vi "VDD over Temp.vi"() -> ()   [LabVIEW 2020]
panel:
  out "Histeresis":dbl[](array[numeric])
  out "VDD down":dbl[](array[numeric])
  out "VDD up":dbl[](array[numeric])
  in  "Thermostream":refnum<visa-resource-name>="GPIB0::11::INSTR"
  out "error out":errorcluster
  in  "Multimetru":refnum<visa-resource-name>="GPIB0::24::INSTR"
  in  "SMU":refnum<visa-resource-name>="GPIB0::1::INSTR"
  in  "error in (no error)":errorcluster
  in  "Temperaturi":dbl[](array[numeric])=[-40.0, 25.0, 80.0, 125.0]
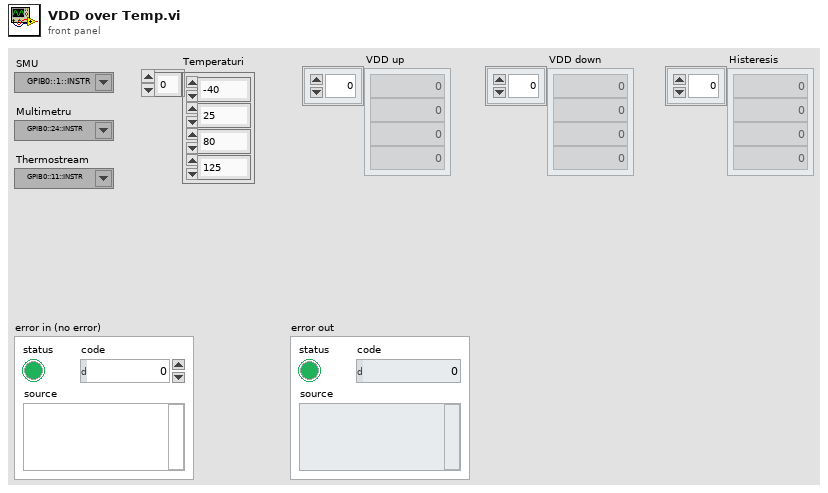
[diagram p1: front panel]
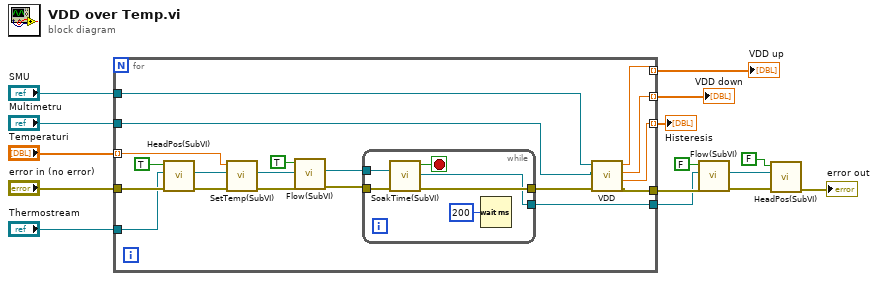
[diagram p0: block diagram]
diagram:
  n1 = for {
    tunnel: "Temperaturi" -> [w31] mode=indexing
    tunnel: "error in (no error)" -> [w34]
    tunnel: "SMU" -> [w22]
    tunnel: "Multimetru" -> [w21]
    tunnel: [w19] -> w10
    tunnel: "Thermostream" -> [w27]
    tunnel: [w23] -> w5
    tunnel: [w18] -> w3 mode=indexing
    tunnel: [w17] -> w2 mode=indexing
    tunnel: [w16] -> w1 mode=indexing
    n2 = call "HeadPos(SubVI).vi"("error in (no error)"=w34, "VISA resource name"=w27, "Checkbox"=TRUE) -> ("error out"=w32:errorcluster, "VISA resource name 2"=w26:refnum<visa-resource-name>)  [unwired: 7 in]
    n3 = call "SetTemp(SubVI).vi"("error in (no error)"=w32, "VISA resource name"=w26, "Temp"=w31) -> ("error out"=w30:errorcluster, "VISA resource name out"=w25:refnum<visa-resource-name>)  [unwired: 7 in]
    n4 = call "Flow(SubVI).vi"("error in (no error)"=w30, "VISA resource name"=w25, "Checkbox"=TRUE) -> ("error out"=w29:errorcluster, "VISA resource name 2"=w24:refnum<visa-resource-name>)  [unwired: 7 in]
    n5 = while {
      tunnel: [w38] -> w20
      tunnel: w29 -> [w39]
      tunnel: w24 -> [w36]
      tunnel: [w35] -> w23
      stop <- w37 stop-if-true
      n6 = call "SoakTime(SubVI).vi"("error in (no error)"=w39, "VISA resource name"=w36) -> ("error out"=w38:errorcluster, "VISA resource name out"=w35:refnum<visa-resource-name>, "soaked?"=w37:bool)  [unwired: 7 in]
      n7 = Wait (ms)(milliseconds to wait=u32 200) -> ()  [unwired: 1 out]
    }
    n8 = call "VDD.vi"("error in (no error)"=w20, "Multimetru"=w21, "SMU"=w22) -> ("error out"=w19:errorcluster, "Histeresis"=w16:dbl, "VDD_min_down"=w17:dbl, "VDD_min_up"=w18:dbl)  [unwired: 5 in]
  }
  "VDD up" <- w3
  "VDD down" <- w2
  "Histeresis" <- w1
  n9 = call "Flow(SubVI).vi"("error in (no error)"=w10, "VISA resource name"=w5, "Checkbox"=FALSE) -> ("error out"=w9:errorcluster, "VISA resource name 2"=w4:refnum<visa-resource-name>)  [unwired: 7 in]
  n10 = call "HeadPos(SubVI).vi"("error in (no error)"=w9, "VISA resource name"=w4, "Checkbox"=FALSE) -> ("error out"=→"error out":errorcluster)  [unwired: 7 in, 1 out]
